vi "INI_Property Files Built With.vi"(7 "File Action":enum16{"Read", "Write"}(ring), 11 "Property Files Built With":cluster{"Scripting":bool, "Private":bool}) -> (3 "Property Files Built With":cluster{"Scripting":bool, "Private":bool})   [LabVIEW 2023]
uses:
  <vilib>/Utility/config.llb/NI_LVConfig.lvlib
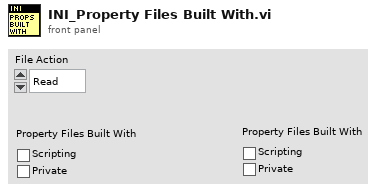
[diagram p1: front panel]
types:
  T1 = typedef "NI_LVConfig.lvlib/Config Data RefNum.ctl" = refnum<k1>
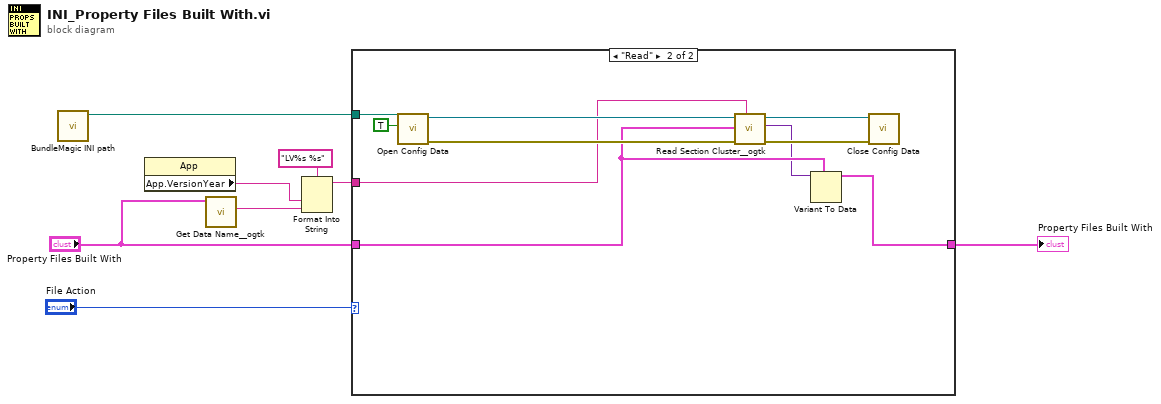
[diagram p0: block diagram]
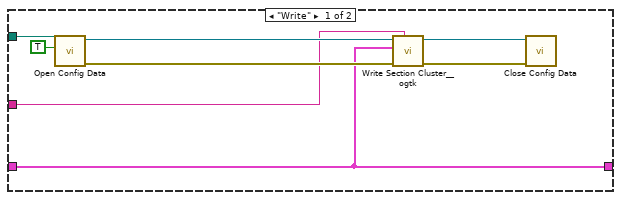
[diagram p2: hidden frame]
diagram:
  n1 = call "BundleMagic INI path.vi"() -> ("appended path"=w8:path)  [unwired: 11 in]
  n2 = property class="App"() -> ("App.VersionYear"=w5:string)  [unwired: 2 in, 2 out]
  n3 = call <userlib>:"Get Data Name__ogtk.vi"("Data"="Property Files Built With") -> ("Data Name"=w4:string)  [unwired: 8 in, 2 out]
  n4 = Format Into String(format string="LV%s %s", w5, w4) -> (resulting string=w1:string)  [unwired: 2 in, 1 out]
  n5 = case shown="\"Read\"" "File Action" {
    tunnel: w8 -> [w16 w22]
    tunnel: "Property Files Built With" -> [w10 w20]
    tunnel: [w10 w18] -> w6
    tunnel: w1 -> [w9 w17]
    frame "Write" {
      n6 = call <vilib>:"Open Config Data.vi"("create file if necessary (T)"=TRUE, "configuration file path"=w16) -> ("error out"=w14:errorcluster, "refnum"=w11:T1)  [unwired: 7 in, 1 out]
      n7 = call <userlib>:"Write Section Cluster__ogtk.vi"("section (optional)"=w9, "error in (no error)"=w14, "Section Formatted Cluster"=w10, "refnum"=w11) -> ("error out"=w13:errorcluster, "dup refnum"=w12:T1)  [unwired: 6 in]
      n8 = call <vilib>:"Close Config Data.vi"("error in (no error)"=w13, "refnum"=w12) -> ()  [unwired: 8 in, 2 out]
    }
    frame "Read" {
      n9 = call <vilib>:"Open Config Data.vi"("create file if necessary (T)"=TRUE, "configuration file path"=w22) -> ("error out"=w24:errorcluster, "refnum"=w26:T1)  [unwired: 7 in, 1 out]
      n10 = call <userlib>:"Read Section Cluster__ogtk.vi"("section (optional)"=w17, "error in (no error)"=w24, "Section Formatted Cluster Type"=w20, "refnum"=w26) -> ("error out"=w23:errorcluster, "Section Formatted Cluster"=w19:variant, "dup refnum"=w25:T1)  [unwired: 3 in, 2 out]
      n11 = Variant To Data(type=w20, Variant=w19) -> (data=w18:cluster{"Scripting":bool, "Private":bool})  [unwired: 1 in, 1 out]
      n12 = call <vilib>:"Close Config Data.vi"("error in (no error)"=w23, "refnum"=w25) -> ()  [unwired: 8 in, 2 out]
    }
  }
  "Property Files Built With" <- w6
